vi "SetOutput.vi"(8 "error in (no error)":errorcluster, 9 "Boolean":bool=TRUE, 10 "Index":i32, 11 "16InOut in":refnum<class "16InOut.lvclass">) -> (0 "error out":errorcluster, 1 "life+1":bool, 3 "16InOut out":refnum<class "16InOut.lvclass">)   [LabVIEW 2019, in "16InOut.lvclass"]
uses:
  16InOut.lvclass
  C:/Users/user/Desktop/204J1/System/Function/IO Folder/IO_Class/IOCard.lvclass
  IOCard.lvclass/IOCard.ctl
  IOCard.lvclass
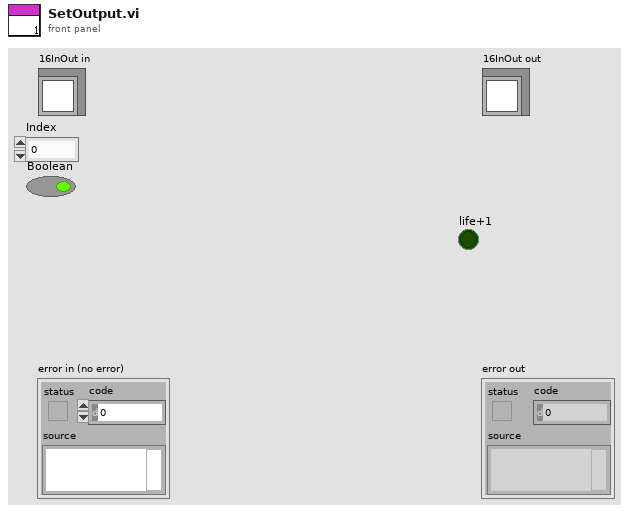
[diagram p1: front panel]
types:
  T1 = typedef "IO Card_Type.ctl" = enum16{"None", "Unidaq32", "6480", "2410C-64", "Zan", "DMC1000B", "16InOut", "Robot", "DMC3600"}
  T2 = cluster{"IO Card Type":T1, "IOType":enum16{"Input", "Output"}, "CardNumber":i32, "ConnectAct":bool, "IP":string}
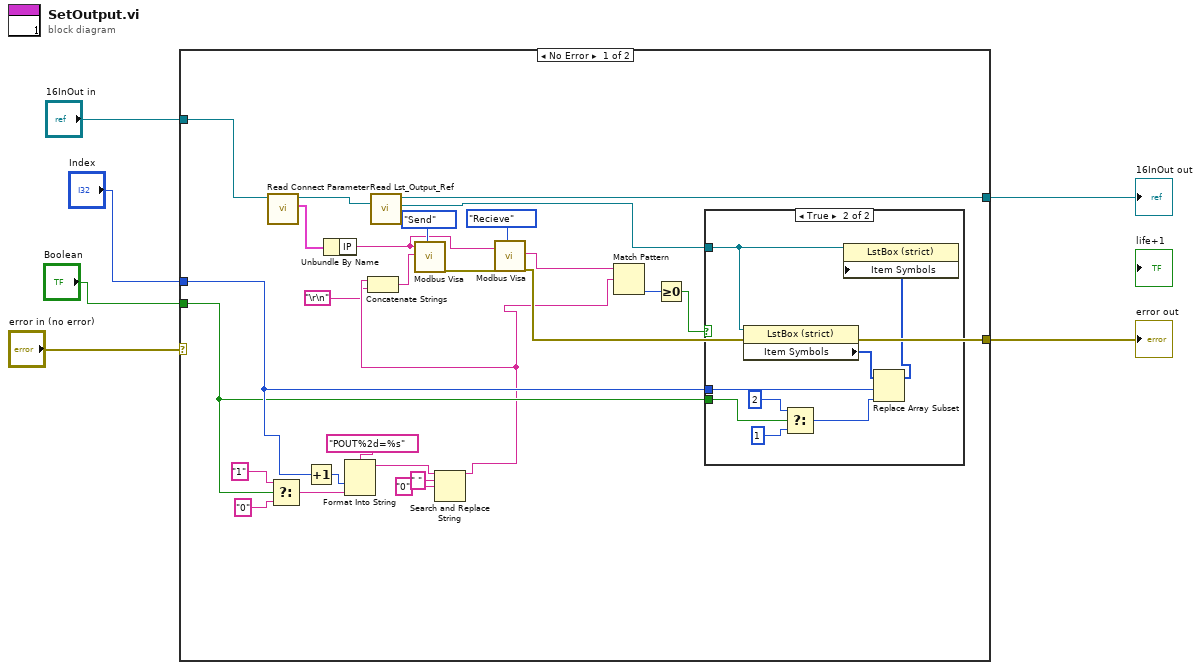
[diagram p0: block diagram]
diagram:
  n1 = case shown="No Error" "error in (no error)" {
    selector: "error in (no error)" -> [_ w41]
    tunnel: [w18 w42] -> w5
    tunnel: "16InOut in" -> [w32 w42]
    tunnel: "Index" -> [w13 _]
    tunnel: "Boolean" -> [w12 _]
    tunnel: [w27 w41] -> w1
    frame No Error {
      n2 = call "Read Connect Parameter.vi"("IOCard in"=w32) -> ("Connect Parameter"=w30:T2, "IOCard out"=w19:refnum<class "16InOut.lvclass">)  [unwired: 8 in, 1 out]
      n3 = Select(t="1", s=w12, f="0") -> (s? t:f=w24:string)
      n4 = Increment(x=w13) -> (x+1=w7:i32)
      n5 = Unbundle By Name(w30) -> ("IP"=w8:string)
      n6 = Format Into String(format string="POUT%2d=%s", w7, w24) -> (resulting string=w22:string)  [unwired: 2 in, 1 out]
      n7 = call-dynamic "Read Lst_Output_Ref.vi"("IOCard in"=w19) -> ("Lst_Output_Ref"=w17:refnum<vi>, "IOCard out"=w18:refnum<class "16InOut.lvclass">)  [unwired: 8 in, 1 out]
      n8 = Search and Replace String(input string=w22, search string=" ", replace string="0" ("replace string (\"\")")) -> (result string=w10:string)  [unwired: 5 in, 3 out]
      n9 = Concatenate Strings(w10, "\r\n") -> (w11:string)
      n10 = call "Modbus Visa.vi"("VISA resource name"=w8, "Cmd"=w11, "VisaAction"=enum16{"Open", "Send", "Recieve", "Close"}."Send") -> ("error out"=w28:errorcluster)  [unwired: 15 in, 1 out]
      n11 = call "Modbus Visa.vi"("VISA resource name"=w8, "error in (no error)"=w28, "VisaAction"=enum16{"Open", "Send", "Recieve", "Close"}."Recieve") -> ("read string"=w16:string, "error out"=w27:errorcluster)  [unwired: 15 in]
      n12 = Match Pattern(string=w16, regular expression=w10) -> (offset past match=w15:i32)  [unwired: 1 in, 3 out]
      n13 = Greater Or Equal To 0?(x=w15) -> (x >= 0?=w14:bool)
      n14 = case shown="True" w14 {
        tunnel: w17 -> [_ w40]
        tunnel: w13 -> [_ w38]
        tunnel: w12 -> [_ w35]
        frame False {
        }
        frame True {
          n15 = property class="LstBox (strict)"(reference=w40) -> ("Item Symbols"=w39:i32[])  [unwired: 1 in, 2 out]
          n16 = Select(t=2, s=w35, f=1) -> (s? t:f=w34:i32)
          n17 = Replace Array Subset(array=w39, new element=w34, index=w38) -> (w33:i32[])
          n18 = property class="LstBox (strict)"(reference=w40, "Item Symbols"=w33) -> ()  [unwired: 1 in, 2 out]
        }
      }
    }
    frame Error {
    }
  }
  "error out" <- w1
  "16InOut out" <- w5
